vi "Facade.vi"(0 "Data In":T5={"Channel 1"=0, "Enable"=TRUE, "Main Switch"=0, "Channel 2"=0, "Channel 3"=0, "Channel 4"=0, "Channel 1"=0, "Channel 5"=0, "Channel 6"=0, "Channel 7"=0, "Channel 8"=0, "Channel 9"=0, "Channel 10"=0, "Channel 11"=0, "Channel 1"=0, "Channel 12"=0, "Channel 13"=0, "Channel 14"=0}, 2 "Display State In":T3, 3 "Container State":T4) -> (6 "Data Out":T5={"Channel 1"=0, "Enable"=TRUE, "Main Switch"=0, "Channel 2"=0, "Channel 3"=0, "Channel 4"=0, "Channel 1"=0, "Channel 5"=0, "Channel 6"=0, "Channel 7"=0, "Channel 8"=0, "Channel 9"=0, "Channel 10"=0, "Channel 11"=0, "Channel 1"=0, "Channel 12"=0, "Channel 13"=0, "Channel 14"=0}, 7 "Display State Out":T3, 8 "Action":T2)   [LabVIEW 2012, in "XControl.xctl"]
uses:
  XControl.xctl
  Data.ctl
  <vilib>/_xctls/Container State.ctl
  State.ctl
  <vilib>/_xctls/Action.ctl
  <vilib>/_xctls/XControlSupport.lvlib
panel:
  in  "Control Panel":T1={"Channel 1"=0, "Enable"=TRUE, "Main Switch"=0, "Channel 2"=0, "Channel 3"=0, "Channel 4"=0, "Channel 1"=0, "Channel 5"=0, "Channel 6"=0, "Channel 7"=0, "Channel 8"=0, "Channel 9"=0, "Channel 10"=0, "Channel 11"=0, "Channel 1"=0, "Channel 12"=0, "Channel 13"=0, "Channel 14"=0}
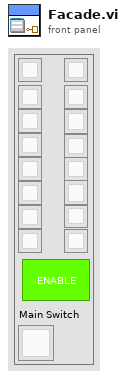
[diagram p1: front panel]
types:
  T1 = cluster{"Channel 1":u8, "Enable":bool, "Main Switch":u8, "Channel 2":u8, "Channel 3":u8, "Channel 4":u8, "Channel 1":u8, "Channel 5":u8, "Channel 6":u8, "Channel 7":u8, "Channel 8":u8, "Channel 9":u8, "Channel 10":u8, "Channel 11":u8, "Channel 1":u8, "Channel 12":u8, "Channel 13":u8, "Channel 14":u8}
  T2 = typedef "XControlSupport.lvlib/Action.ctl" = cluster{"Data Changed?":bool, "State Changed?":bool, "Action Name":string}
  T3 = typedef "XControl.xctl/State.ctl" = cluster{"Numeric":dbl}
  T4 = typedef "XControlSupport.lvlib/Container State.ctl" = cluster{"Indicator?":bool, "Run Mode?":bool, " Refnum":refnum<vi>}
  T5 = typedef "XControl.xctl/Data.ctl" = cluster{"Channel 1":u8, "Enable":bool, "Main Switch":u8, "Channel 2":u8, "Channel 3":u8, "Channel 4":u8, "Channel 1":u8, "Channel 5":u8, "Channel 6":u8, "Channel 7":u8, "Channel 8":u8, "Channel 9":u8, "Channel 10":u8, "Channel 11":u8, "Channel 1":u8, "Channel 12":u8, "Channel 13":u8, "Channel 14":u8}
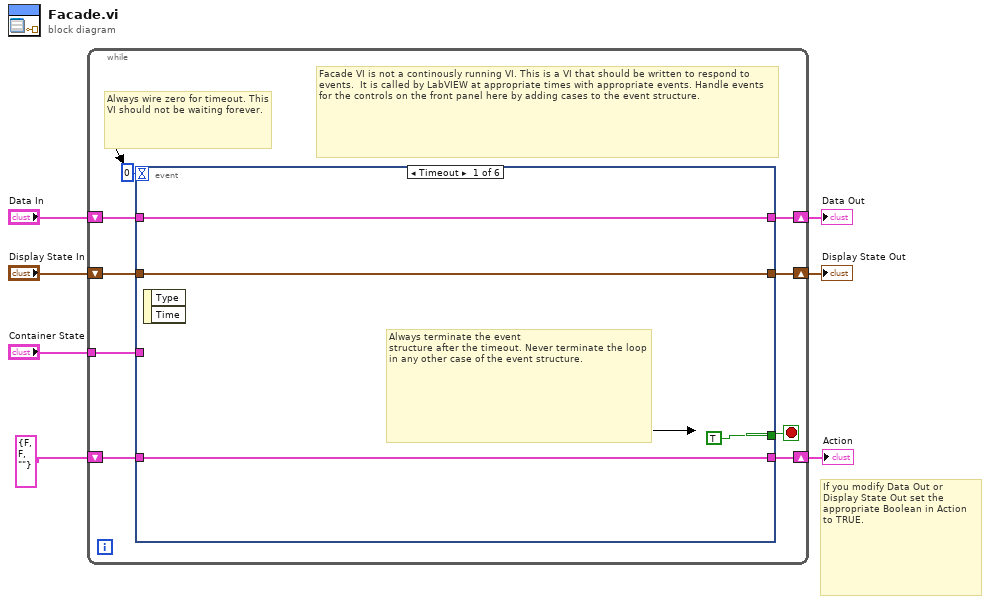
[diagram p0: block diagram]
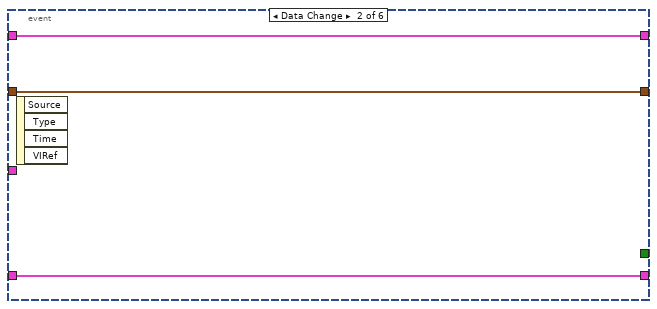
[diagram p2: hidden frame]
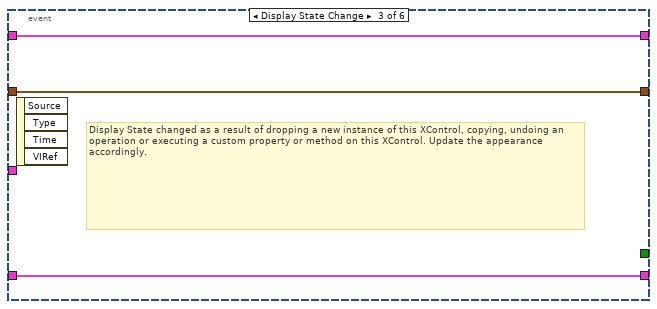
[diagram p3: hidden frame]
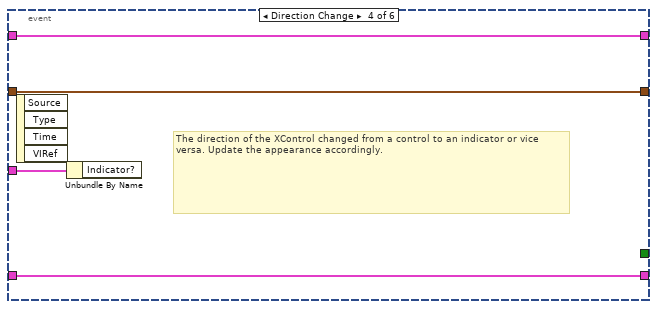
[diagram p4: hidden frame]
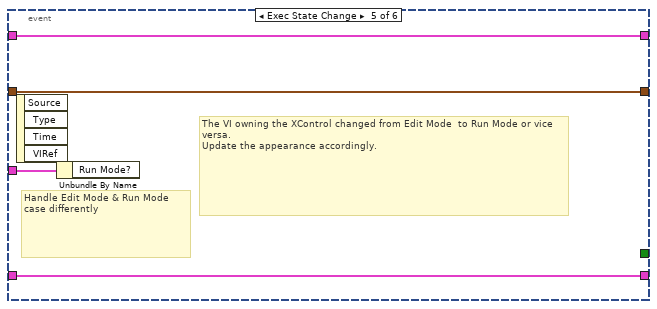
[diagram p5: hidden frame]
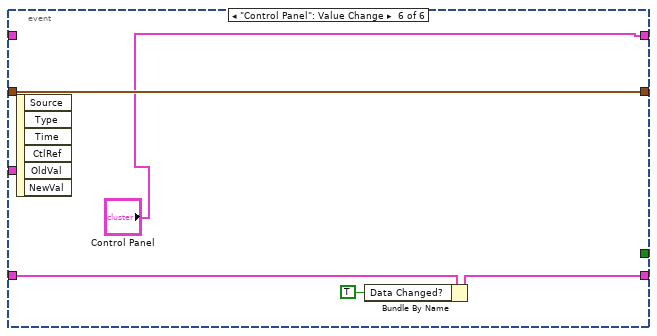
[diagram p6: hidden frame]
diagram:
  # "If you modify Data Out or\nDisplay State Out set the\nappropriate Boolean in Action\nto TRUE."
  n1 = while {
    shift-right: [w15] -> w4
    shift-left: "Display State In" -> [w16]
    tunnel: "Container State" -> [w12]
    shift-right: [w10] -> w7
    shift-left: "Data In" -> [w11]
    shift-right: [w8] -> w2
    shift-left: T2 {"Data Changed?"=FALSE, "State Changed?"=FALSE, "Action Name"=""} ("Action") -> [w9]
    stop <- w14 stop-if-true
    # "Facade VI is not a continously running VI. This is a VI that should be written to respond to events.  It is called by LabVIEW at appropriate times with appropriate events. Handle events for the controls on the front panel here by adding cases to the event structure."
    # "Always wire zero for timeout. This\nVI should not be waiting forever."
    n2 = event shown="[0] Timeout" {
      selector: _ -> [_ _ _ _ _ _]
      dyn-events: _ -> [_ _ _ _ _ _]
      timeout: 0 -> [_ _ _ _ _ _]
      tunnel: w16 -> [w18 w23 w26 w29 w33 w39]
      tunnel: [w18 w23 w26 w29 w33 w39] -> w15
      tunnel: [TRUE _ _ _ _ _] -> w14
      tunnel: w12 -> [_ _ _ w30 w34 _]
      tunnel: w11 -> [w17 w21 w25 w28 w32 _]
      tunnel: [w17 w21 w25 w28 w32 "Control Panel"] -> w10
      tunnel: [w19 w22 w24 w27 w31 w37] -> w8
      tunnel: w9 -> [w19 w22 w24 w27 w31 w38]
      event Timeout {
        # "Always terminate the event\nstructure after the timeout. Never terminate the loop in any other case of the event structure."
        n3 = event-data() -> ()  [unwired: 1 in, 2 out]
      }
      event Data Change {
        n4 = event-data() -> ()  [unwired: 1 in, 4 out]
      }
      event Display State Change {
        # "Display State changed as a result of dropping a new instance of this XControl, copying, undoing an operation or executing a custom property or method on this XControl. Update the appearance accordingly."
        n5 = event-data() -> ()  [unwired: 1 in, 4 out]
      }
      event Direction Change {
        # "The direction of the XControl changed from a control to an indicator or vice versa. Update the appearance accordingly."
        n6 = event-data() -> ()  [unwired: 1 in, 4 out]
        n7 = Unbundle By Name(w30) -> ()  [unwired: 1 out]
      }
      event Exec State Change {
        # "The VI owning the XControl changed from Edit Mode  to Run Mode or vice versa.\nUpdate the appearance accordingly."
        # "Handle Edit Mode & Run Mode\ncase differently"
        n8 = event-data() -> ()  [unwired: 1 in, 4 out]
        n9 = Unbundle By Name(w34) -> ()  [unwired: 1 out]
      }
      event "Control Panel": Value Change {
        n10 = event-data() -> ()  [unwired: 1 in, 6 out]
        n11 = Bundle By Name(cluster=w38, "Data Changed?"=TRUE) -> (w37:T2)
      }
    }
  }
  "Display State Out" <- w4
  "Data Out" <- w7
  "Action" <- w2
